vi "Graph data.vi"(8 "error in (no error)":errorcluster, 10 "Graph data":dbl, 11 "Generador de funciones in":refnum<class "Generador de funciones.lvclass">) -> (0 "error out":errorcluster, 3 "Generador de funciones out":refnum<class "Generador de funciones.lvclass">)   [LabVIEW 2019, in "Generador de funciones.lvlib" / "Generador de funciones.lvclass"]
uses:
  Generador de funciones.lvclass
  Generador de funciones.lvclass/Generador de funciones.ctl
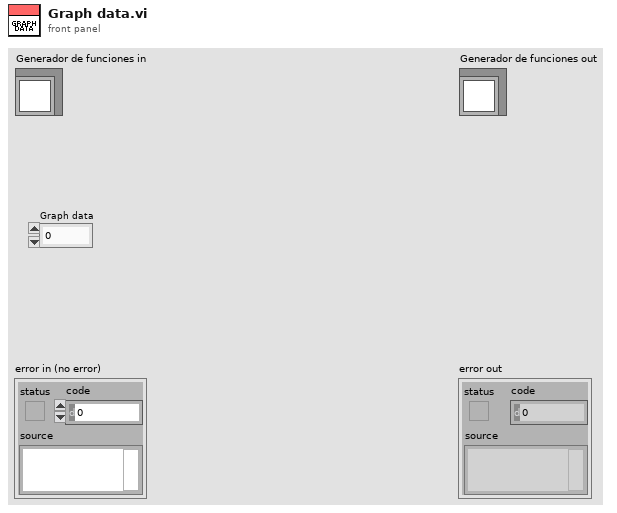
[diagram p1: front panel]
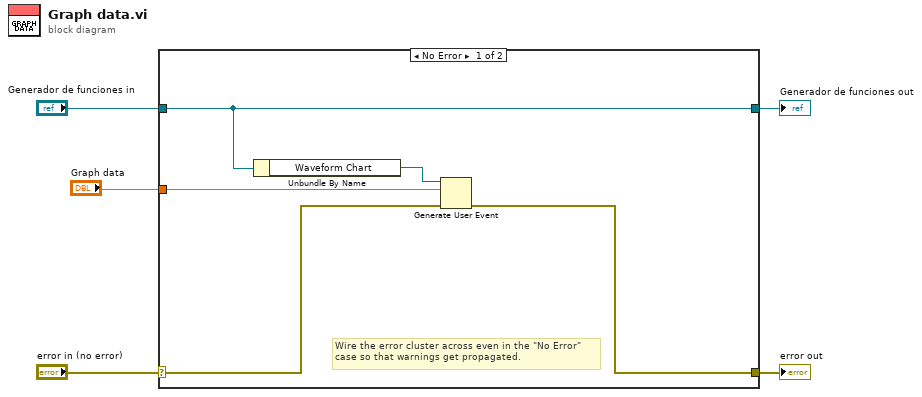
[diagram p0: block diagram]
diagram:
  n1 = case shown="No Error" "error in (no error)" {
    selector: "error in (no error)" -> [w8 w12]
    tunnel: [w7 w12] -> w4
    tunnel: [w10 w11] -> w2
    tunnel: "Generador de funciones in" -> [w10 w11]
    tunnel: "Graph data" -> [w6 _]
    frame No Error {
      # "Wire the error cluster across even in the \"No Error\"\ncase so that warnings get propagated."
      n2 = Unbundle By Name(w10) -> ("Waveform Chart"=w9:refnum<user-event>)
      n3 = Generate User Event(user event=w9, event data cluster=w6, error in=w8) -> (error out=w7:errorcluster)  [unwired: 1 in, 1 out]
    }
    frame Error {
    }
  }
  "error out" <- w4
  "Generador de funciones out" <- w2
